vi "EstructuraSequenceEjemplo.vi"() -> ()   [LabVIEW 2022 SP3]
panel:
  out "Tank":i8(slide) scale=0.0..100.0
  # "Llenado y vaciado de un tanque con Sequence"
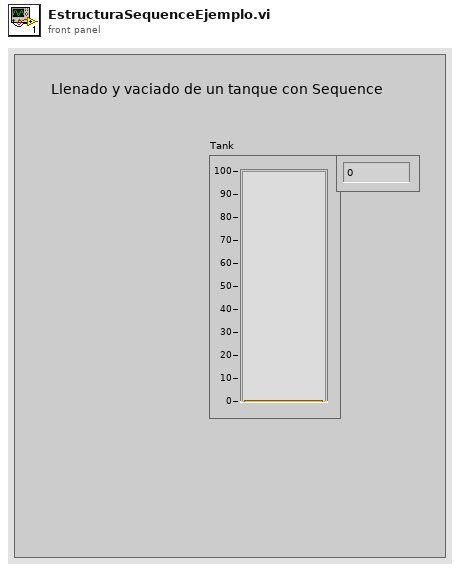
[diagram p1: front panel]
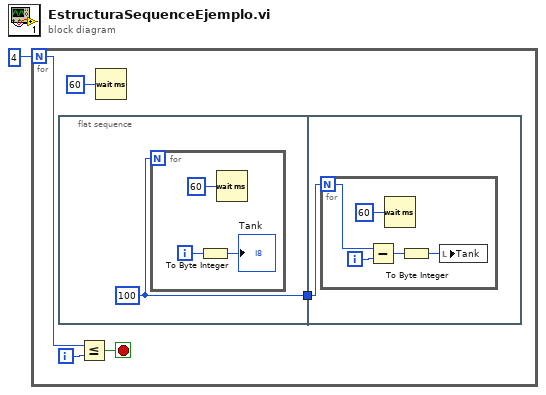
[diagram p0: block diagram]
diagram:
  n1 = for {
    N: 4 -> [w5]
    i -> [w4]
    stop <- w3 stop-if-true
    n2 = flat-sequence {
      tunnel: [w7] -> w6
      tunnel: w6 -> [w11]
      frame #0 {
        w7 = 100
        n3 = for {
          N: w7 -> [_]
          i -> [w9]
          n4 = To Byte Integer(number=w9) -> (8bit integer=→"Tank":i8)
          n5 = Wait (ms)(milliseconds to wait=u32 60) -> ()  [unwired: 1 out]
        }
      }
      frame #1 {
        n6 = for {
          N: w11 -> [w15]
          i -> [w14]
          n7 = Subtract(x=w15, y=w14) -> (x-y=w13:i32)
          n8 = Wait (ms)(milliseconds to wait=u32 60) -> ()  [unwired: 1 out]
          n9 = To Byte Integer(number=w13) -> (8bit integer=w12:i8)
          n10 = local write "Tank"(w12) -> ()
        }
      }
    }
    n11 = Less Or Equal?(x=w5, y=w4) -> (x <= y?=w3:bool)
    n12 = Wait (ms)(milliseconds to wait=u32 60) -> ()  [unwired: 1 out]
  }
